vi "Tag.GetChannelRefs.vi"(7 "Access":T1=enum."Write", 8 "error in (no error)":errorcluster, 10 "Dependent Node Ref":T2 format="%.0x", 11 "Section Ref in":T2 format="%.0x") -> (0 "error out":errorcluster, 2 "Array":T3[](array[typedef]) format="%.0x", 3 "Section Ref out":T2 format="%.0x")   [LabVIEW 2019, in "OPC UA Client Addon System Explorer.lvlib"]
uses:
  OPC UA Client Addon System Explorer.lvlib
  <vilib>/NI VeriStand/Custom Device API/Custom Device Item Ref.ctl
  <vilib>/NI VeriStand/Custom Device API/Data Reference.ctl
  <vilib>/NI VeriStand/Custom Device API/Data Access Type.ctl
  <vilib>/NI VeriStand/Custom Device API/Custom Device API.lvlib
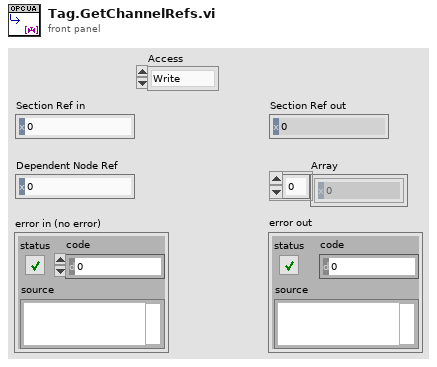
[diagram p1: front panel]
types:
  T1 = typedef "Custom Device API.lvlib/Data Access Type.ctl" = enum16{"Read", "Write"}
  T2 = typedef "Custom Device API.lvlib/Custom Device Item Ref.ctl" = u64
  T3 = typedef "Custom Device API.lvlib/Data Reference.ctl" = i32
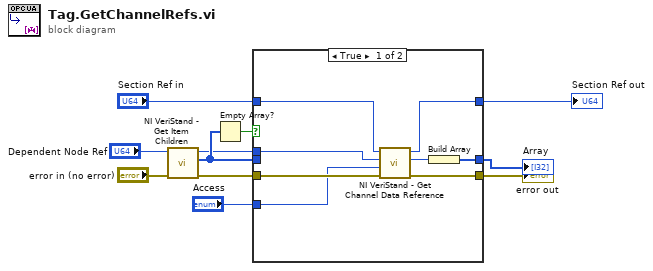
[diagram p0: block diagram]
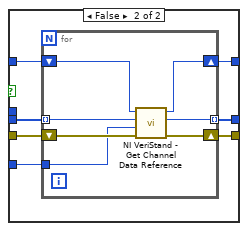
[diagram p2: hidden frame]
diagram:
  n1 = call <vilib>:"NI VeriStand - Get Item Children.vi"("error in (no error)"="error in (no error)", "Item Ref in"="Dependent Node Ref") -> ("error out"=w7:errorcluster, "Child Refs"=w11:T2[], "Item Ref out"=w9:T2)  [unwired: 6 in, 1 out]
  n2 = Empty Array?(array=w11) -> (empty?=w10:bool)
  n3 = case shown="True" w10 {
    tunnel: [w19 w26] -> w2
    tunnel: "Section Ref in" -> [w18 w25]
    tunnel: [w13 w22] -> w4
    tunnel: [w16 w24] -> w5
    tunnel: w7 -> [w15 w23]
    tunnel: w9 -> [w14 _]
    tunnel: w11 -> [_ w21]
    tunnel: "Access" -> [w12 w20]
    frame True {
      n4 = call <vilib>:"NI VeriStand - Get Channel Data Reference.vi"("error in (no error)"=w15, "Access"=w12, "Channel Ref in"=w14, "Device Ref in"=w18) -> ("error out"=w19:errorcluster, "Channel Data Reference"=w17:T3, "Device Ref out"=w16:T2)  [unwired: 5 in]
      n5 = Build Array(w17) -> (w13:T3[])
    }
    frame False {
      n6 = for {
        tunnel: w21 -> [w29] mode=indexing
        tunnel: [w28] -> w22 mode=indexing
        shift-right: [w33] -> w26
        shift-left: w23 -> [w30]
        shift-right: [w31] -> w24
        shift-left: w25 -> [w32]
        tunnel: w20 -> [w27]
        n7 = call <vilib>:"NI VeriStand - Get Channel Data Reference.vi"("error in (no error)"=w30, "Access"=w27, "Channel Ref in"=w29, "Device Ref in"=w32) -> ("error out"=w33:errorcluster, "Channel Data Reference"=w28:T3, "Device Ref out"=w31:T2)  [unwired: 5 in]
      }
    }
  }
  "Section Ref out" <- w5
  "Array" <- w4
  "error out" <- w2
